vi "PID Veering.vi"(6 "Deviation":dbl, 7 "Current Distance":dbl=15.0 format="%#_13g", 8 "error in (no error)":errorcluster, 11 "Refnum's":T1={"Gyro"="Gyro", "Mtr 1"="LeftMtr", "Mtr 2"="RightMtr"}) -> (0 "error out":errorcluster)   [LabVIEW 2017]
uses:
  <vilib>/addons/control/pid/pid.llb/PID (DBL).vi
  <vilib>/addons/control/pid/NI_PID_pid.lvlib
panel:
  out "Waveform Graph":dbl[](graph)
  in  "V-D":dbl format="%#_13g"
  in  "V-I":dbl format="%#_13g"
  in  "V-P":dbl=0.06 format="%#_13g"
  in  "D-D":dbl format="%#_13g"
  in  "D-I":dbl format="%#_13g"
  in  "D-P":dbl=0.0007 format="%#_13g"
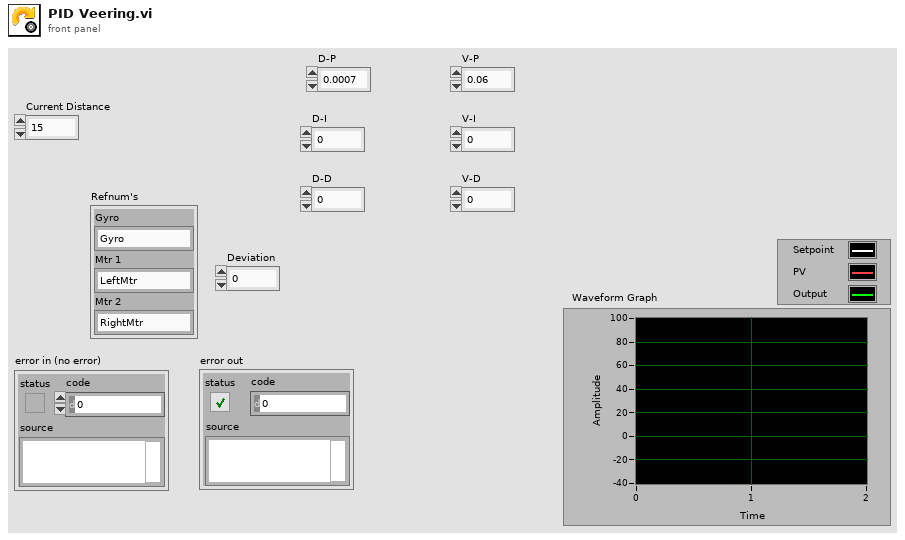
[diagram p1: front panel]
types:
  T1 = cluster{"Gyro":string, "Mtr 1":string, "Mtr 2":string}
  T2 = typedef "WPI_MotorControlDeviceRef.ctl" = cluster{"DeviceStatus":errorcluster, "Type":T3, "PWM":cluster{"PWM Channel":T4, "DeadBand":T5}, "CAN":cluster{"Device Number":u8, "SetOutput VI Ref":variant, "GetOutput VI Ref":variant, "Enable VI Ref":variant, "Disable VI Ref":variant, "Data":variant}, "Invert":bool, "DIO PWM":cluster{"PWM \"Enable\" Channel":T4, "DIOChannel":T6, "PWM Rate":dbl}}
  T3 = typedef "WPI_MotorControlType.ctl" = enum16{"PWM", "CAN", "DIO PWM"}
  T4 = typedef "FPGA_DIOPWMChannel.ctl" = enum8{"PWM 0", "PWM 1", "PWM 2", "PWM 3", "PWM 4", "PWM 5", "PWM 6", "PWM 7", "PWM 8", "PWM 9", "PWM MXP 0", "PWM MXP 1", "PWM MXP 2", "PWM MXP 3", "PWM MXP 4", "PWM MXP 5", "PWM MXP 6", "PWM MXP 7", "PWM MXP 8", "PWM MXP 9", "Invalid"}
  T5 = typedef "WPI_PWMDeadband.ctl" = cluster{"Name":string, "maxPositivePwm":i32, "minPositivePwm":i32, "centerPwm":i32, "maxNegativePwm":i32, "minNegativePwm":i32, "angularRange":u16}
  T6 = typedef "FPGA_DIOChannel.ctl" = enum8{"DIO 0", "DIO 1", "DIO 2", "DIO 3", "DIO 4", "DIO 5", "DIO 6", "DIO 7", "DIO 8", "DIO 9", "DIO MXP 0", "DIO MXP 1", "DIO MXP 2", "DIO MXP 3", "DIO MXP 4", "DIO MXP 5", "DIO MXP 6", "DIO MXP 7", "DIO MXP 8", "DIO MXP 9", "DIO MXP 10", "DIO MXP 11", "DIO MXP 12", "DIO MXP 13", "DIO MXP 14", "DIO MXP 15", "SPI Port CS1", "SPI Port CS2", "SPI Port CS3", "SPI Port MISO", "SPI Port MOSI", "Invalid"}
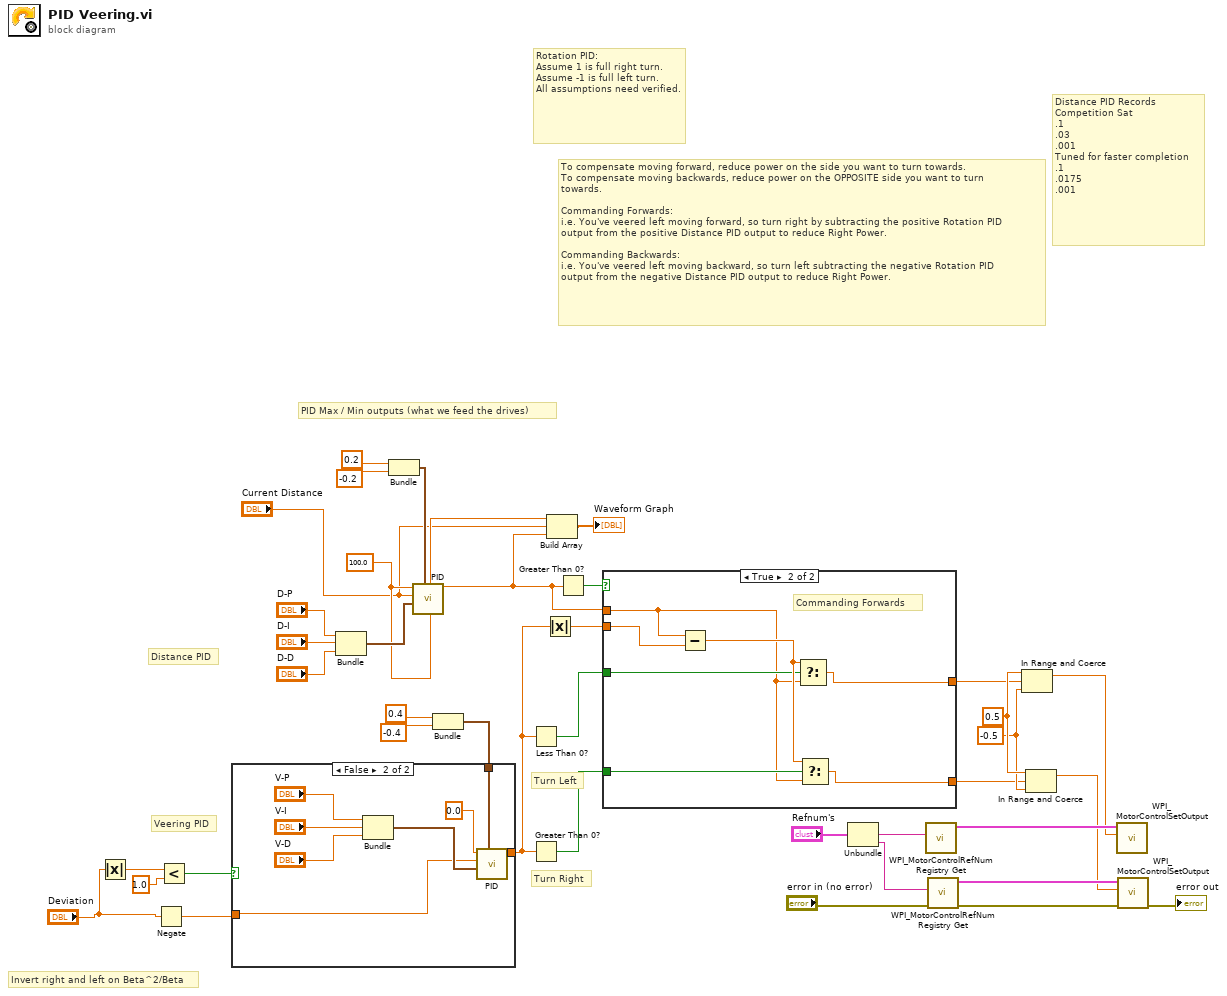
[diagram p0: block diagram]
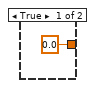
[diagram p2: hidden frame]
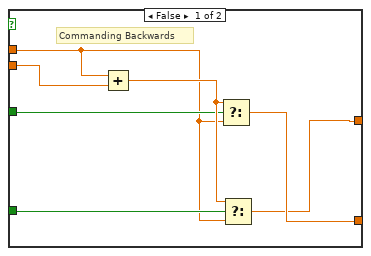
[diagram p3: hidden frame]
diagram:
  w12 = 100.0 ("setpoint")
  w27 = -0.5
  w28 = 0.5
  # "Veering PID"
  # "Distance PID"
  # "Distance PID Records\nCompetition Sat\n.1\n.03\n.001\nTuned for faster completion\n.1\n.0175\n.001"
  # "Invert right and left on Beta^2/Beta"
  # "Turn Right"
  # "Turn Left"
  # "To compensate moving forward, reduce power on the side you want to turn towards.\nTo compensate moving backwards, reduce power on the OPPOSITE side you want to turn\ntowards.\n\nCommanding Forwards:\ni.e. You've veered left moving forward, so turn right by subtracting the positive Rotation PID\noutput from the positive Distance PID output to reduce Right Power.\n\nCommanding Backwards:\ni.e. You've veered left moving backward, so turn left subtracting the negative Rotation PID \noutput from the negative Distance PID output to reduce Right Power."
  # "PID Max / Min outputs (what we feed the drives)"
  # "Rotation PID:\nAssume 1 is full right turn.\nAssume -1 is full left turn.\nAll assumptions need verified."
  n1 = Absolute Value(x="Deviation") -> (abs(x)=w8:dbl)
  n2 = Negate(x="Deviation") -> (-x=w1:dbl)
  n3 = Less?(x=w8, y=1.0) -> (x < y?=w7:bool)
  n4 = Bundle("D-P"="D-P", "D-I"="D-I", "D-D"="D-D") -> (w31:cluster{"D-P":dbl, "D-I":dbl, "D-D":dbl})  [unwired: 1 in]
  n5 = Bundle(0.2, -0.2) -> (w30:cluster{dbl, dbl})  [unwired: 1 in]
  n6 = call-poly <vilib>:"PID.vi"("output range"=w30, "PID gains"=w31, "process variable"="Current Distance", "setpoint"=w12) -> ("output"=w10:dbl)  [unwired: 6 in, 1 out]
  n7 = Bundle(0.4, -0.4) -> (w4:cluster{dbl, dbl})  [unwired: 1 in]
  n8 = case shown="False" w7 {
    tunnel: w4 -> [_ w43]
    tunnel: [0.0 ("output") w42] -> w21
    tunnel: w1 -> [_ w40]
    frame True {
    }
    frame False {
      n9 = Bundle("V-P"="V-P", "V-I"="V-I", "V-D"="V-D") -> (w44:cluster{"V-P":dbl, "V-I":dbl, "V-D":dbl})  [unwired: 1 in]
      n10 = call-poly <vilib>:"PID.vi"("output range"=w43, "PID gains"=w44, "process variable"=w40, "setpoint"=0.0) -> ("output"=w42:dbl)  [unwired: 6 in, 1 out]
    }
  }
  n11 = Less Than 0?(x=w21) -> (x < 0?=w23:bool)
  n12 = Greater Than 0?(x=w21) -> (x > 0?=w22:bool)
  n13 = Absolute Value(x=w21) -> (abs(x)=w26:dbl)
  n14 = Build Array(w12, "Current Distance", w10) -> (→"Waveform Graph":dbl[])
  n15 = Greater Than 0?(x=w10) -> (x > 0?=w29:bool)
  n16 = case shown="True" w29 {
    tunnel: w26 -> [w51 w61]
    tunnel: w10 -> [w48 w55]
    tunnel: [w50 w59] -> w25
    tunnel: [w49 w58] -> w24
    tunnel: w23 -> [w53 w57]
    tunnel: w22 -> [w52 w56]
    frame False {
      # "Commanding Backwards"
      n17 = Add(x=w48, y=w51) -> (x+y=w54:dbl)
      n18 = Select(t=w54, s=w53, f=w48) -> (s? t:f=w50:dbl)
      n19 = Select(t=w54, s=w52, f=w48) -> (s? t:f=w49:dbl)
    }
    frame True {
      # "Commanding Forwards"
      n20 = Subtract(x=w55, y=w61) -> (x-y=w60:dbl)
      n21 = Select(t=w60, s=w57, f=w55) -> (s? t:f=w58:dbl)
      n22 = Select(t=w60, s=w56, f=w55) -> (s? t:f=w59:dbl)
    }
  }
  n23 = Unbundle("Refnum's") -> ("Mtr 1"=w38:string, "Mtr 2"=w37:string)  [unwired: 1 out]
  n24 = call <vilib>:"WPI_MotorControlRefNum Registry Get.vi"("refnum name"=w38) -> ("MotorControlDevRef"=w18:T2)  [unwired: 9 in, 1 out]
  n25 = call <vilib>:"WPI_MotorControlRefNum Registry Get.vi"("error in (no error)"="error in (no error)", "refnum name"=w37) -> ("error out"=w13:errorcluster, "MotorControlDevRef"=w19:T2)  [unwired: 8 in]
  n26 = In Range and Coerce(upper limit=w28, x=w24, lower limit=w27) -> (coerced(x)=w17:dbl)  [unwired: 1 out]
  n27 = In Range and Coerce(upper limit=w28, x=w25, lower limit=w27) -> (coerced(x)=w16:dbl)  [unwired: 1 out]
  n28 = call <vilib>:"WPI_MotorControlSetOutput.vi"("Output"=w17, "MotorControlDevRef"=w18) -> ()  [unwired: 7 in, 3 out]
  n29 = call <vilib>:"WPI_MotorControlSetOutput.vi"("error in (no error)"=w13, "Output"=w16, "MotorControlDevRef"=w19) -> ("error out"=→"error out":errorcluster)  [unwired: 6 in, 2 out]
